vi "Example_GSF.vi"() -> ()   [LabVIEW 2021]
uses:
  Main/Ver_2/Config_File_Paths_v2.ctl
  <instrlib>/Zurich Instruments LabOne/Public/Modules/ziTypeModEnum.ctl
  <instrlib>/Zurich Instruments LabOne/Zurich Instruments LabOne.lvlib
panel:
  out "Front":cluster{"Time":dbl[], "Y":dbl[]}(graph)
  out "Front":dbl[](array[numeric])
  out "Back Sum":dbl[](array[numeric])
  in  "error in":errorcluster
  out "ZI DATA3":cluster{"Time":dbl[], "R":dbl[]}(graph)
  out "ZI DATA0":cluster{"Time":dbl[], "R":dbl[]}(graph)
  out "ZI DATA3 OUTPUT":cluster{"Time":dbl[], "R":dbl[]}
  out "ZI DATA0 OUTPUT":cluster{"Time":dbl[], "R":dbl[]}
  out "error out":errorcluster
  in  "Config files paths":T1={"ZI config file (.ini)"="Config_Ver_2\\GSF_Zurich_params.ini", "Keithley config file (.ini)"="Config_Ver_2\\Keithley_params.ini", "DAQ config file (.ini)"="Config_Ver_2\\GSF_pulse_sequence_DAQ.ini"}
  in  "keithley":refnum<visa-resource-name>="KEITHLEY"
  in  "AI duration (ms)":i32=100
  in  "Address":string="DEV714"
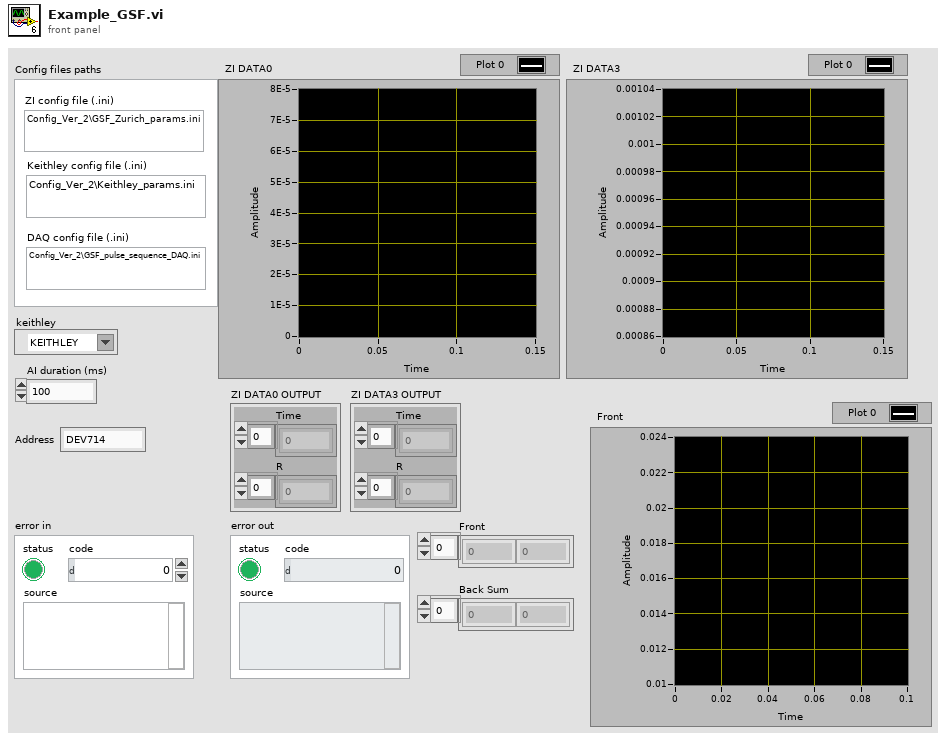
[diagram p1: front panel]
types:
  T1 = typedef "Config_File_Paths_v2.ctl" = cluster{"ZI config file (.ini)":string, "Keithley config file (.ini)":string, "DAQ config file (.ini)":string}
  T2 = typedef "Zurich Instruments LabOne.lvlib/ziTypeModEnum.ctl" = u16
  T3 = typedef "Zurich Instruments LabOne.lvlib/ziTypeHandle.ctl" = cluster{"handleValid":bool, "Conn":u64, "Path Prefix":string, "Handle":u64, "Clockbase(s)":dbl, "Connected":bool}
  T4 = typedef "Zurich Instruments LabOne.lvlib/ziTypeModHandle.ctl" = cluster{"handleValid":bool, "Conn":u64, "ModHandle":u64, "moduleID":string, "Path Prefix":string}
  T5 = cluster{"Handle Out":T3, "ModHandle Out":T4, "keithley":refnum<visa-resource-name>}
  T6 = typedef "Resources_v2.ctl" = cluster{"ZI Handle":T3, "ZI ModHandle":T4, "VISA Keithley":refnum<visa-resource-name>}
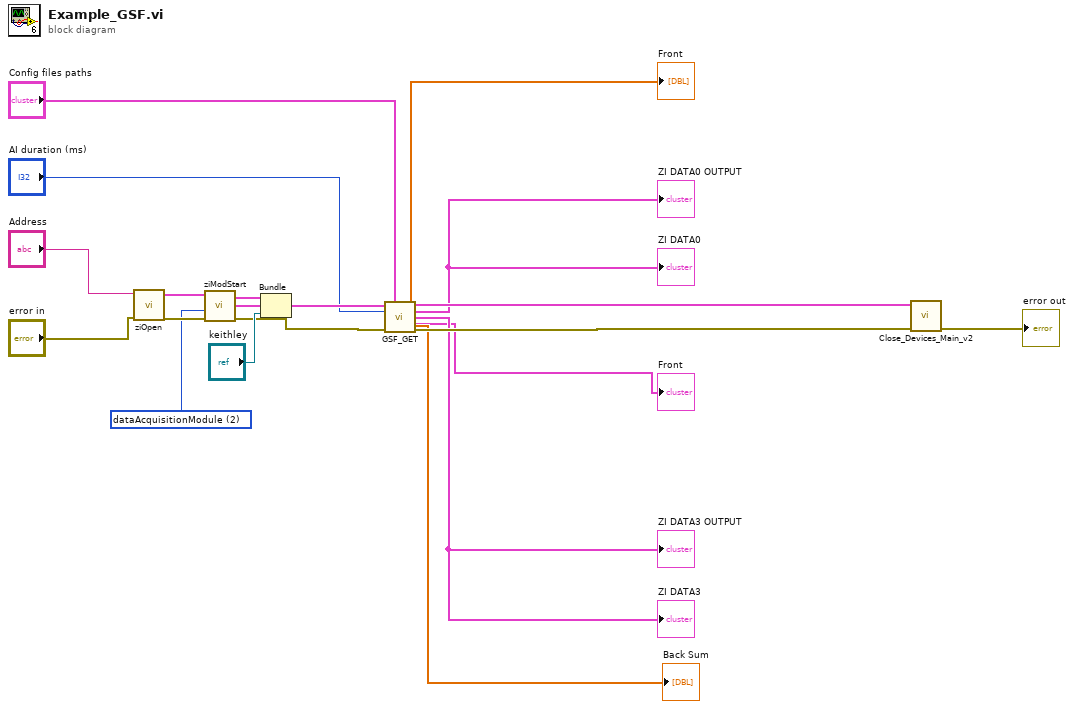
[diagram p0: block diagram]
diagram:
  w17 = T2 2 items=["sweep", "scopeModule", "dataAcquisitionModule", "pidAdvisor", "awgModule", "impedanceModule", "multiDeviceSyncModule", "zoomFFT", "trigger", "deviceSettings", "record", "precompensationAdvisor"] ("module Id")
  n1 = call <instrlib>:"ziOpen.vi"("Error In"="error in", "Address"="Address") -> ("Error Out"=w18:errorcluster, "HandleOut"=w19:T3)  [unwired: 2 in, 1 out]
  n2 = call <instrlib>:"ziModStart.vi"("Error In"=w18, "module Id"=w17, "Handle In"=w19) -> ("Error Out"=w11:errorcluster, "ModHandle Out"=w15:T4, "Handle Out"=w16:T3)  [unwired: 6 in]
  n3 = Bundle("Handle Out"=w16, "ModHandle Out"=w15, "keithley"="keithley") -> (w14:T5)  [unwired: 1 in]
  n4 = call "GSF_GET.vi"("Resources in"=w14, "Config files paths"="Config files paths", "AI duration (ms)"="AI duration (ms)", "error in"=w11) -> ("Front"=→"Front":dbl[], "Resources out"=w9:T6, "ZI DATA0 OUTPUT"=→"ZI DATA0 OUTPUT" →"ZI DATA0":cluster{"Time":dbl[], "R":dbl[]}, "ZI DATA3 OUTPUT"=→"ZI DATA3 OUTPUT" →"ZI DATA3":cluster{"Time":dbl[], "R":dbl[]}, "Front Data"=→"Front":cluster{"Time":dbl[], "Y":dbl[]}, "Back Sum"=→"Back Sum":dbl[], "error out"=w8:errorcluster)  [unwired: 4 in, 1 out]
  n5 = call "Close_Devices_Main_v2.vi"("error in"=w8, "Resources"=w9) -> ("error out"=→"error out":errorcluster)  [unwired: 9 in]
